vi "Get UDP Reference.vi"(8 "error in (no error)":errorcluster) -> (0 "error out":errorcluster, 3 "UDP Network Connection":refnum<k16>)   [LabVIEW 2016, in "Client.lvlib" / "Client.lvclass"]
uses:
  Client.lvclass
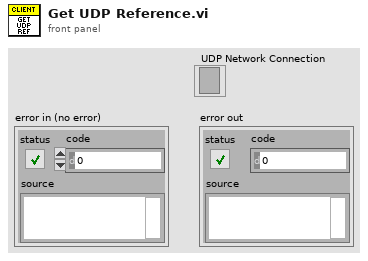
[diagram p1: front panel]
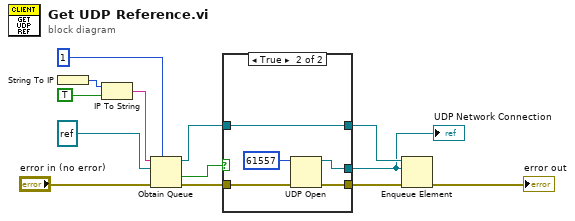
[diagram p0: block diagram]
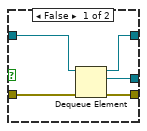
[diagram p2: hidden frame]
diagram:
  n1 = String To IP() -> (0:w9:u32)  [unwired: 1 in]
  n2 = IP To String(1:TRUE ("dot notation? (F)"), 2:w9) -> (0:w7:string)
  n3 = Obtain Queue(max queue size (-1, unlimited)=1, name (unnamed)=w7, element data type=refnum<k16> refnum ("connection ID"), error in (no error)="error in (no error)") -> (queue out=w5:refnum<queue>, created new?=w6:bool, error out=w11:errorcluster)  [unwired: 1 in]
  n4 = case shown="True" w6 {
    tunnel: [w15 w23] -> w2
    tunnel: [w14 w22] -> w12
    tunnel: w11 -> [w18 w20]
    tunnel: w5 -> [w17 w19]
    tunnel: [w16 w19] -> w3
    frame False {
      n5 = Dequeue Element(queue=w17, error in (no error)=w18) -> (queue out=w16:refnum<queue>, element=w15:refnum<k16>, error out=w14:errorcluster)  [unwired: 1 in, 1 out]
    }
    frame True {
      n6 = UDP Open(8:w20, 11:u16 61557 ("local port")) -> (port=w23:refnum<k16>, 0:w22:errorcluster)  [unwired: 3 in, 1 out]
    }
  }
  "UDP Network Connection" <- w2
  n7 = Enqueue Element(queue=w3, element=w2, error in (no error)=w12) -> (error out=→"error out":errorcluster)  [unwired: 1 in, 2 out]
